vi "Pipe Var Intf - Test Pipe Create Speed.vi"() -> ()   [LabVIEW 2020, in "GOLPI library.lvlib"]
uses:
  GOLPI library.lvlib
panel:
  out "x/y":dbl
  out "error out":errorcluster
  in  "pipe name":string="\\\\.\\Pipe\\MyNamedPipe"
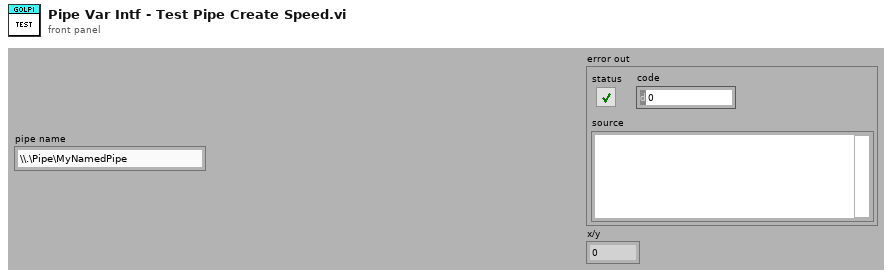
[diagram p1: front panel]
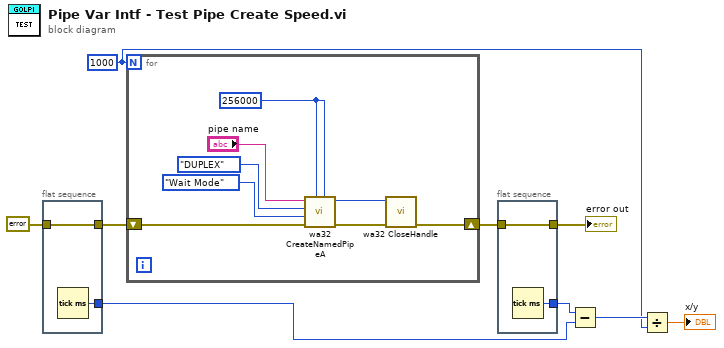
[diagram p0: block diagram]
diagram:
  w2 = 1000
  n1 = flat-sequence {
    tunnel: [w11] -> w8
    tunnel: errorcluster {"status"=FALSE, "code"=0, "source"=""} ("error out") -> [w11]
    tunnel: [w10] -> w4
    frame #0 {
      n2 = Tick Count (ms)() -> (millisecond timer value=w10:u32)
    }
  }
  n3 = for {
    N: w2 -> [_]
    shift-right: [w13] -> w7
    shift-left: w8 -> [w12]
    w16 = u32 256000 ("outBufferSize (256k)")
    n4 = call "wa32 CreateNamedPipeA.vi"("inBufferSize (256k)"=w16, "outBufferSize (256k)"=w16, "error in"=w12, "pipe mode"=enum16{"Wait Mode", "No Wait Mode"}."Wait Mode", "open mode"=enum16{"INBOUND", "OUTBOUND", "DUPLEX"}."DUPLEX", "file path"="pipe name") -> ("error out"=w15:errorcluster, "handle"=w14:i32)  [unwired: 4 in]
    n5 = call "wa32 CloseHandle.vi"("error in"=w15, "handle"=w14) -> ("error out"=w13:errorcluster)  [unwired: 9 in]
  }
  n6 = flat-sequence {
    tunnel: [w21] -> w6
    tunnel: w7 -> [w21]
    tunnel: [w20] -> w5
    frame #0 {
      n7 = Tick Count (ms)() -> (millisecond timer value=w20:u32)
    }
  }
  n8 = Subtract(x=w5, y=w4) -> (x-y=w3:u32)
  n9 = Divide(x=w3, y=w2) -> (x/y=→"x/y":dbl)
  "error out" <- w6
